vi "find_circles test.vi"() -> ()   [LabVIEW 2023]
uses:
  find_circles parameters.ctl
  Vision.lvlib
panel:
  in  "Field of View":cluster{"fieldOfViewX":sgl, "fieldOfViewY":sgl}={"fieldOfViewX"=1.4, "fieldOfViewY"=1.048}
  in  "find_circles parameters":T1={"minRadius"=0.1, "maxRadius"=1.0, "houghGradientParam1"=100, "houghGradientParam2"=50}
  out "Circles":T2(array[cluster])
  out "Number of Circles":i32
  in  "File Path":path
  out "error out":errorcluster
  out "Image":T3(plugin-control)
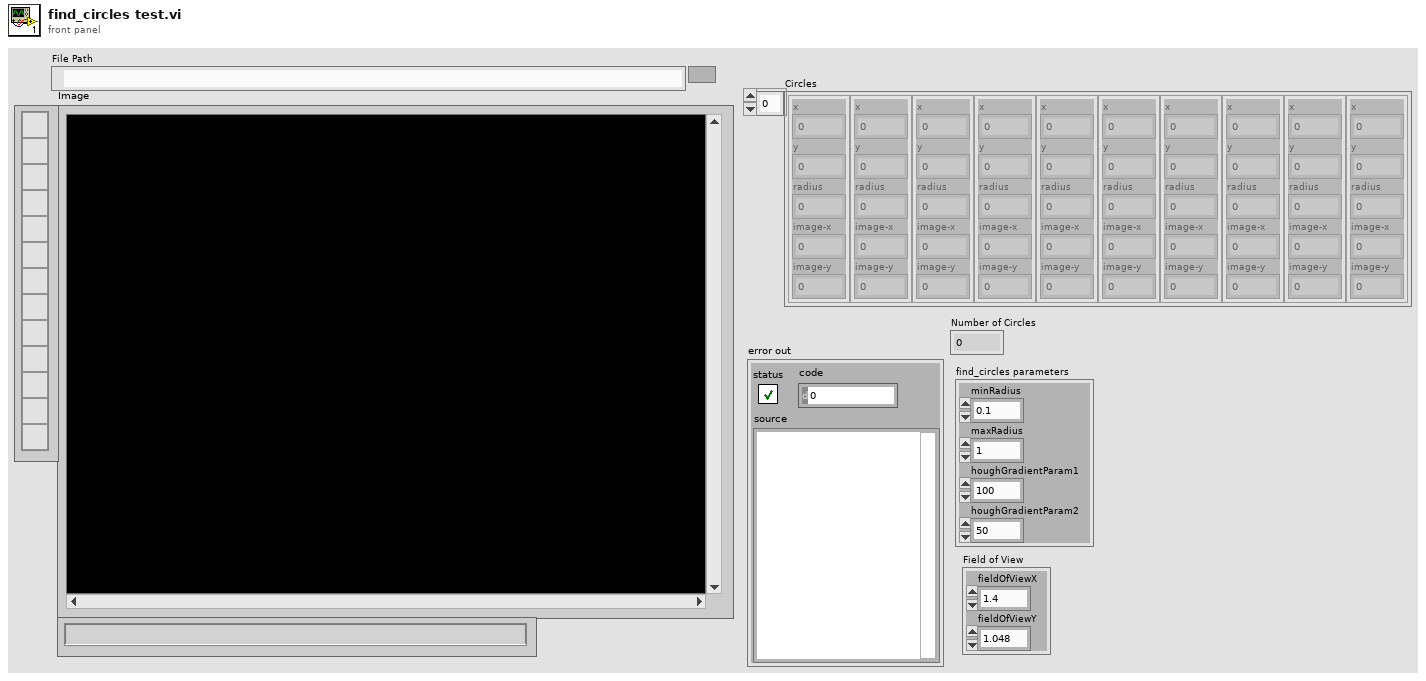
[diagram p1: front panel]
types:
  T1 = typedef "Vision.lvlib/find_circles parameters.ctl" = cluster{"minRadius":sgl, "maxRadius":sgl, "houghGradientParam1":i32, "houghGradientParam2":i32}
  T2 = cluster{"x":dbl, "y":dbl, "radius":dbl, "image-x":dbl, "image-y":dbl}[]
  T3 = typedef "IMAQ Image.ctl" = refnum<image>
  T4 = cluster{"Left":i32, "Top":i32, "Right":i32, "Bottom":i32}
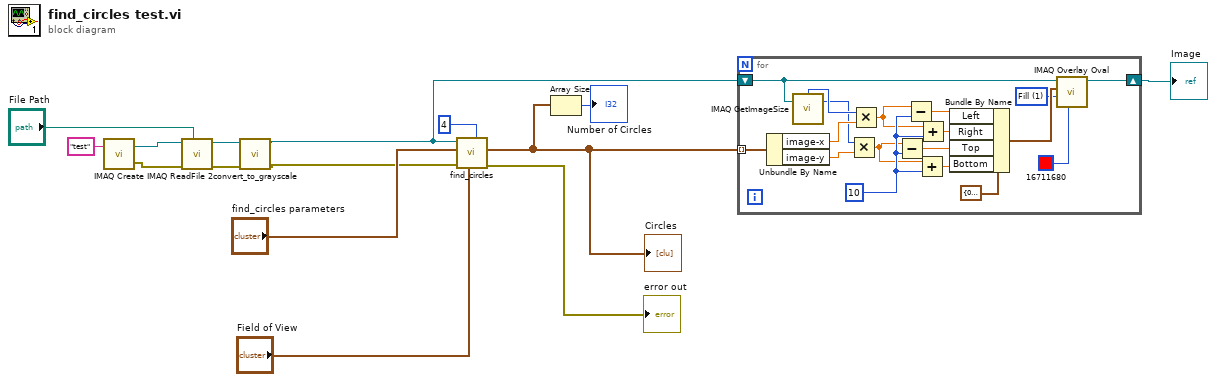
[diagram p0: block diagram]
diagram:
  n1 = call "IMAQ Create"("Image Name"="test") -> ("New Image"=w15:T3, "error out"=w13:errorcluster)  [unwired: 4 in]
  n2 = call "IMAQ ReadFile 2"("File Path"="File Path", "error in (no error)"=w13, "Image"=w15) -> ("error out"=w2:errorcluster, "Image Out"=w4:T3)  [unwired: 4 in, 3 out]
  n3 = call "convert_to_grayscale.vi"("error in (no error)"=w2, "Image in"=w4) -> ("error out"=w1:errorcluster, "Image out"=w3:T3)  [unwired: 8 in]
  n4 = call "find_circles.vi"("shrinkFactor"=4 ("Shrink Factor"), "Field of View"="Field of View", "error in"=w1, "find_circles parameters"="find_circles parameters", "Image"=w3) -> ("error out"=→"error out":errorcluster, "Circles"=w6:T2)  [unwired: 5 in]
  "Circles" <- w6
  n5 = Array Size(array=w6) -> (size(s)=→"Number of Circles":i32)
  n6 = for {
    tunnel: w6 -> [w33] mode=indexing
    shift-right: [w17] -> w5
    shift-left: w3 -> [w28]
    w16 = u32 1 items=["Frame", "Fill"] ("Drawing Mode (Frame)")
    w21 = 10
    n7 = Unbundle By Name(w33) -> ("image-x"=w32:dbl, "image-y"=w30:dbl)
    n8 = call "IMAQ GetImageSize"("Image"=w28) -> ("Y Resolution"=w29:i32, "X Resolution"=w31:i32)  [unwired: 3 in, 1 out]
    n9 = Multiply(x=w29, y=w30) -> (x*y=w20:dbl)
    n10 = Multiply(x=w31, y=w32) -> (x*y=w19:dbl)
    n11 = Subtract(x=w20, y=w21) -> (x-y=w22:dbl)
    n12 = Subtract(x=w19, y=w21) -> (x-y=w23:dbl)
    n13 = Add(x=w20, y=w21) -> (x+y=w24:dbl)
    n14 = Add(x=w19, y=w21) -> (x+y=w25:dbl)
    n15 = Bundle By Name(cluster=T4 {"Left"=0, "Top"=0, "Right"=0, "Bottom"=0} ("Bounding Rectangle"), "Left"=w23, "Right"=w25, "Top"=w22, "Bottom"=w24) -> (w18:T4)
    n16 = call "IMAQ Overlay Oval"("Color"=u32 16711680, "Drawing Mode (Frame)"=w16, "Bounding Rectangle"=w18, "Image"=w28) -> ("Image Out"=w17:T3)  [unwired: 6 in, 1 out]
  }
  "Image" <- w5
